vi "host - network - RT (separate).vi"() -> ()   [LabVIEW 2011]
uses:
  Output - Cluster b2g2.ctl
  Input - Cluster b2g2.ctl
panel:
  in  "Pfad":path=path "C:/National Instruments/Logs"
  out "FS-2 [l]":sgl format="%#.2g"
  out "FS-1 [l]":sgl format="%#.2g"
  out "pH-Wert":cluster{"pHS-1":dbl}(graph)
  out "pHS-1":dbl
  in  "Interval [s]":u32=1 min=1 step=1
  in  "Interval [ms]":u32=10 min=10 step=1
  in  "Output - Cluster":T1 {"TS-5 [°C]" format="%#.2g"; "pHS-1 [pH]" format="%.2g"; "TS-4 [°C]" format="%#.2g"; "FS-2 [l]" format="%.2g"; "FS-1 [l]" format="%.2g"; "DS-1 [bar]" format="%#.2g"; "DFS-1 [l/min]" format="%#.2g"; "FS-3 [l]" format="%.2g"; "DFS-1 [dl]" format="%.0g"}
  in  "Host Log":bool
  in  "P-5":bool
  in  "P-5 Drehzahl [%]":u8
  out "T-2 Min!":bool
  out "T-2 Max!":bool
  out "T-1 Min!":bool
  out "T-1 Max!":bool
  in  "Zulauf Füllstandsüberwachung":bool
  in  "MR Füllstandsüberwachung":bool
  out "Heizung":bool
  in  "Temp Soll [°C]":sgl min=0 max=100 step=0.1 format="%.1g"
  in  "Hysterese [°C]":sgl=0.1 min=0.1 max=10 step=0.1 format="%.1g"
  out "Temperaturregelung":cluster{"Temp Soll":sgl, "TS-4":dbl, i32}(graph)
  in  "Temperaturregelung":bool
  out "Temp Ist [°C]":sgl format="%.2g"
  in  "HS-1":bool
  out "Fütterung":bool
  out "Rezikulation":bool
  in  "Zulauf":bool
  out "Dosierung Fertig":bool
  out "Bereits dosiert":sgl
  out "MIN!":bool
  out "MAX!":bool
  out "Pumpendrehzahl":u8
  in  "Dosiermenge [l]":sgl format="%.1g"
  out "Volumen [l]":sgl format="%.1f"
  out "Durchfluss [l/min]":sgl format="%.2f"
  in  "Dosiergeschwindigkeit [l/min]":sgl format="%.1g"
  out "Dosierung":T2(graph)
  in  "Dosierung":bool
  out "Überdruckregelung":cluster{"Druck Soll":sgl, "DS-1":dbl, dbl}(graph)
  in  "Druck Soll [bar]":sgl min=0 max=10 step=0.1 format="%.1g"
  in  "D":sgl
  in  "I":sgl
  in  "P":sgl
  in  "Füllstand Soll [l]":sgl min=0 max=5 step=0.1 format="%.1g"
  in  "D":sgl
  in  "I":sgl
  in  "P":sgl
  in  "Überdruckregelung":bool
  out "Füllstandsregelung":cluster{"Füllstand Soll":sgl, "FS-3":dbl, dbl}(graph)
  in  "Füllstandsregulierung":bool
  in  "P-4":bool
  in  "P-4 Drehzahl  [%]":u8
  in  "Target Log":bool
  in  "V-15  [%]":u8 max=100 step=1
  in  "Input - Cluster":T3 {"Dosiergeschw. [l/min]" format="%.2g"; "Füllstand  P" max=100 step=1 format="%#_3g"; "P-4 Drehzahl [%]" max=100 step=1 format="%#_3g"}
  in  "V-13 [%]":u8 caption="V-13" max=100 step=1
  out "Füllstand Ist":sgl format="%#.2g"
  out "Druck Ist":sgl format="%#.2g"
  in  "stop":bool
  # "Dosierung"
  # "Handsteuerungen"
  # "Max: 4l\nMin: 1l"
  # "T-1"
  # "T-2"
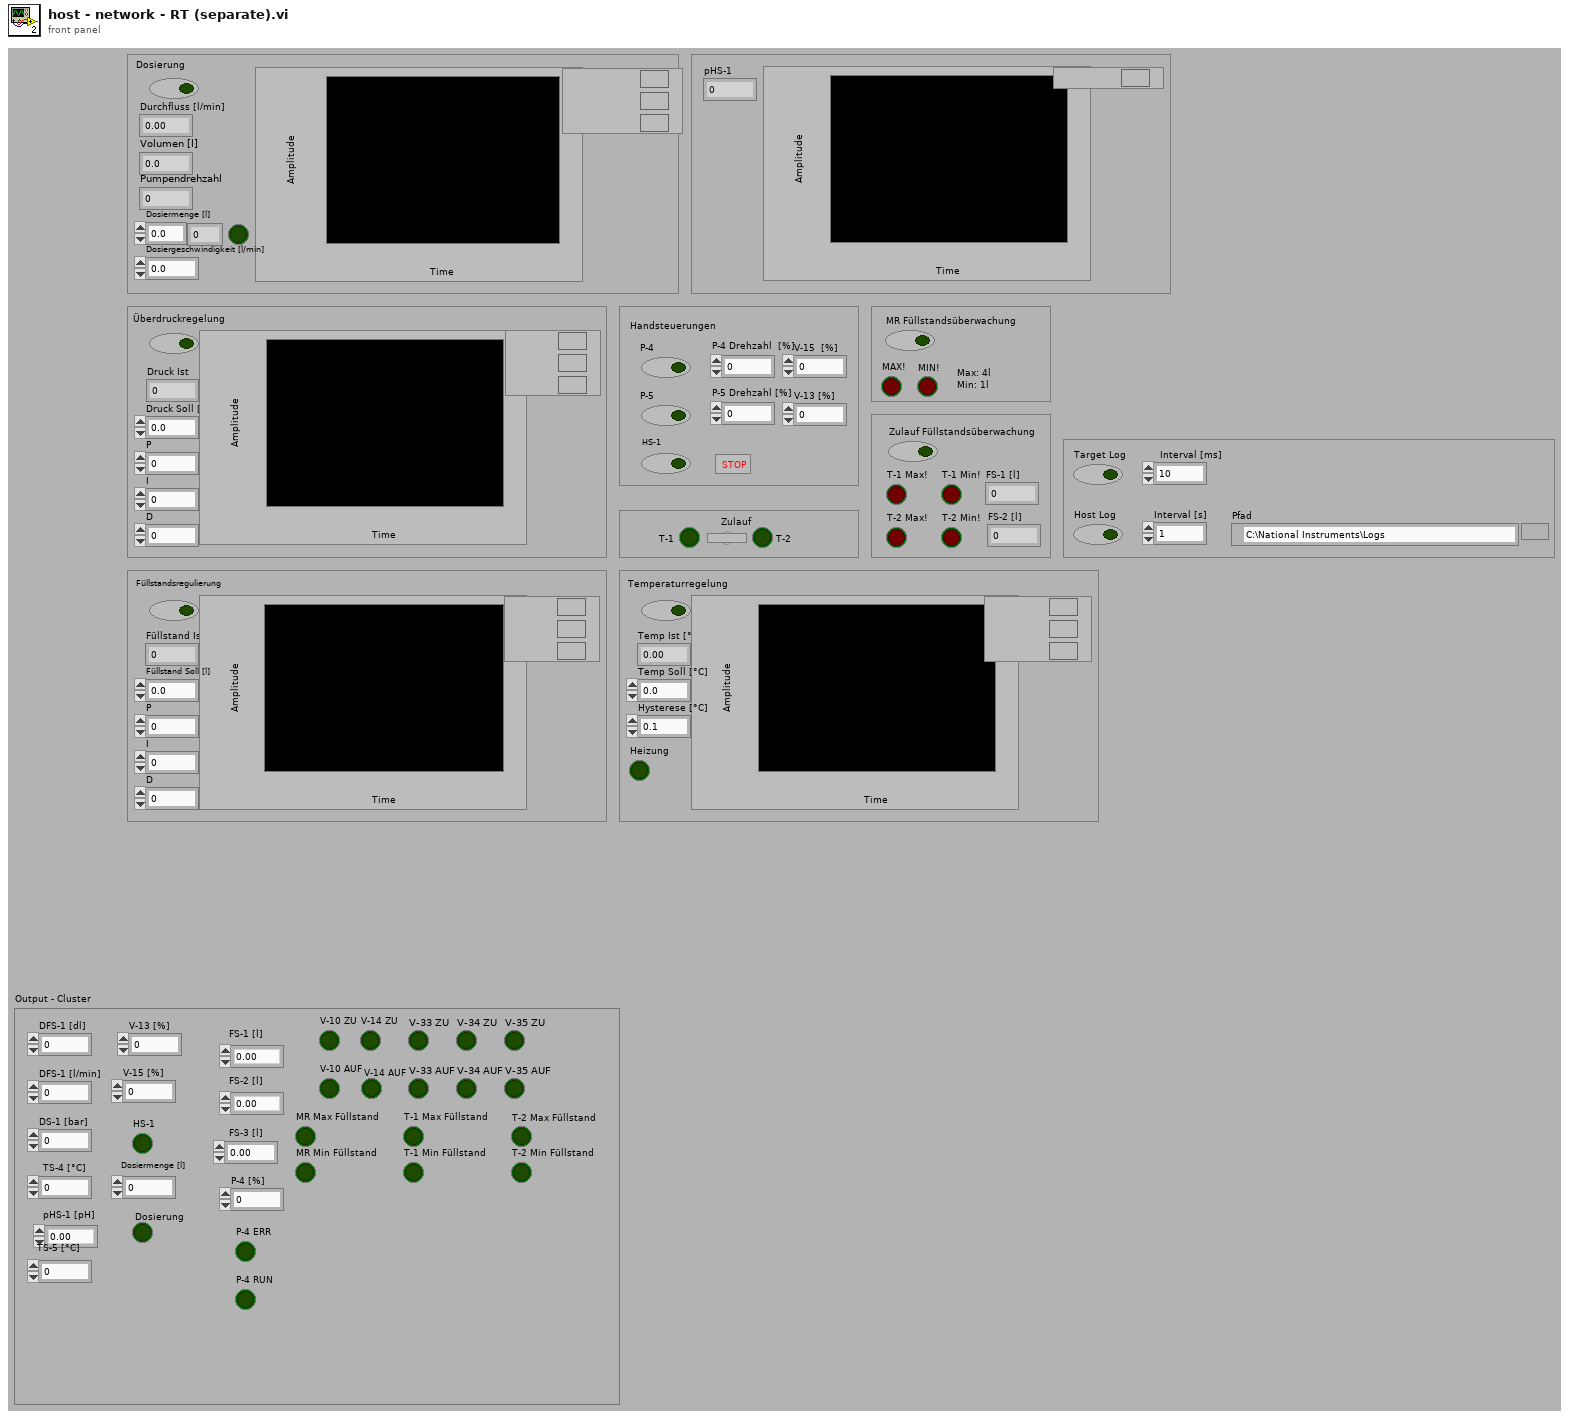
[diagram p1: front panel]
types:
  T1 = typedef "Output - Cluster b2g2.ctl" = cluster{"DFS-1 [dl]":u64, "FS-3 [l]":dbl, "DFS-1 [l/min]":dbl, "DS-1 [bar]":dbl, "V-10 ZU":bool, "V-14 ZU":bool, "FS-1 [l]":dbl, "FS-2 [l]":dbl, "TS-4 [°C]":dbl, "HS-1":bool, "V-13 [%]":u8, "V-15 [%]":u8, "P-4 [%]":u8, "Dosierung":bool, "MR Max Füllstand":bool, "MR Min Füllstand":bool, "Dosiermenge [l]":sgl, "V-14 AUF":bool, "V-10 AUF":bool, "T-1 Max Füllstand":bool, "T-1 Min Füllstand":bool, "T-2 Max Füllstand":bool, "T-2 Min Füllstand":bool, "pHS-1 [pH]":dbl, "P-4 RUN":bool, "V-33 AUF":bool, "V-33 ZU":bool, "V-34 AUF":bool, "V-34 ZU":bool, "P-4 ERR":bool, "TS-5 [°C]":dbl, "V-35 AUF":bool, "V-35 ZU":bool}
  T2 = cluster{"Dosiergeschwindigkeit [l/min]":sgl, "DFS-1 Durchfluss":dbl, dbl}
  T3 = typedef "Input - Cluster b2g2.ctl" = cluster{"V-13 [%]":u8, "V-15 [%]":u8, "Log-Target":bool, "P-4":bool, "P-4 Drehzahl [%]":u8, "Temperaturregelung":bool, "Überdruckregelung":bool, "Füllstandsregulierung":bool, "V-10":bool, "Log-Host":bool, "V-14":bool, "HS-1":bool, "Füllstand  P":sgl, "Füllstand I":sgl, "Füllstand D":sgl, "Füllstand Soll [l]":sgl, "Druck  P":sgl, "Druck I":sgl, "Druck D":sgl, "Druck Soll [bar]":sgl, "Temp Soll [°C]":sgl, "Dosierung":bool, "Dosiermenge [l]":sgl, "Dosiergeschw. [l/min]":sgl, "Tank":bool, "Hysterese [°C]":sgl, "MR Füllstandsüberwachung":bool, "Tank Füllstandsüberwachung":bool, "Log Target [ms]":u32, "Log Host [s]":u32, "Zirkulation EIN [min]":u8, "Zirkulation AUS [min]":u8, "Zirkulation":bool, "V-33":bool, "V-34":bool, "V-35":bool}
  T4 = enum8{"Enabled", "Disabled", "Disabled and Grayed Out"}
  T5 = enum16{"open", "replace", "create", "open or create", "replace or create", "replace or create with confirmation"}
  T6 = cluster{"Temp Soll [°C]":sgl, "TS-4 [°C]":dbl, i32}
  T7 = cluster{"Druck Soll [bar]":sgl, "DS-1 [bar]":dbl, dbl}
  T8 = cluster{"Füllstand Soll [l]":sgl, "FS-3 [l]":dbl, dbl}
  T9 = cluster{"Dosiergeschwindigkeit [l/min]":sgl, "DFS-1 [l/min]":dbl, dbl}
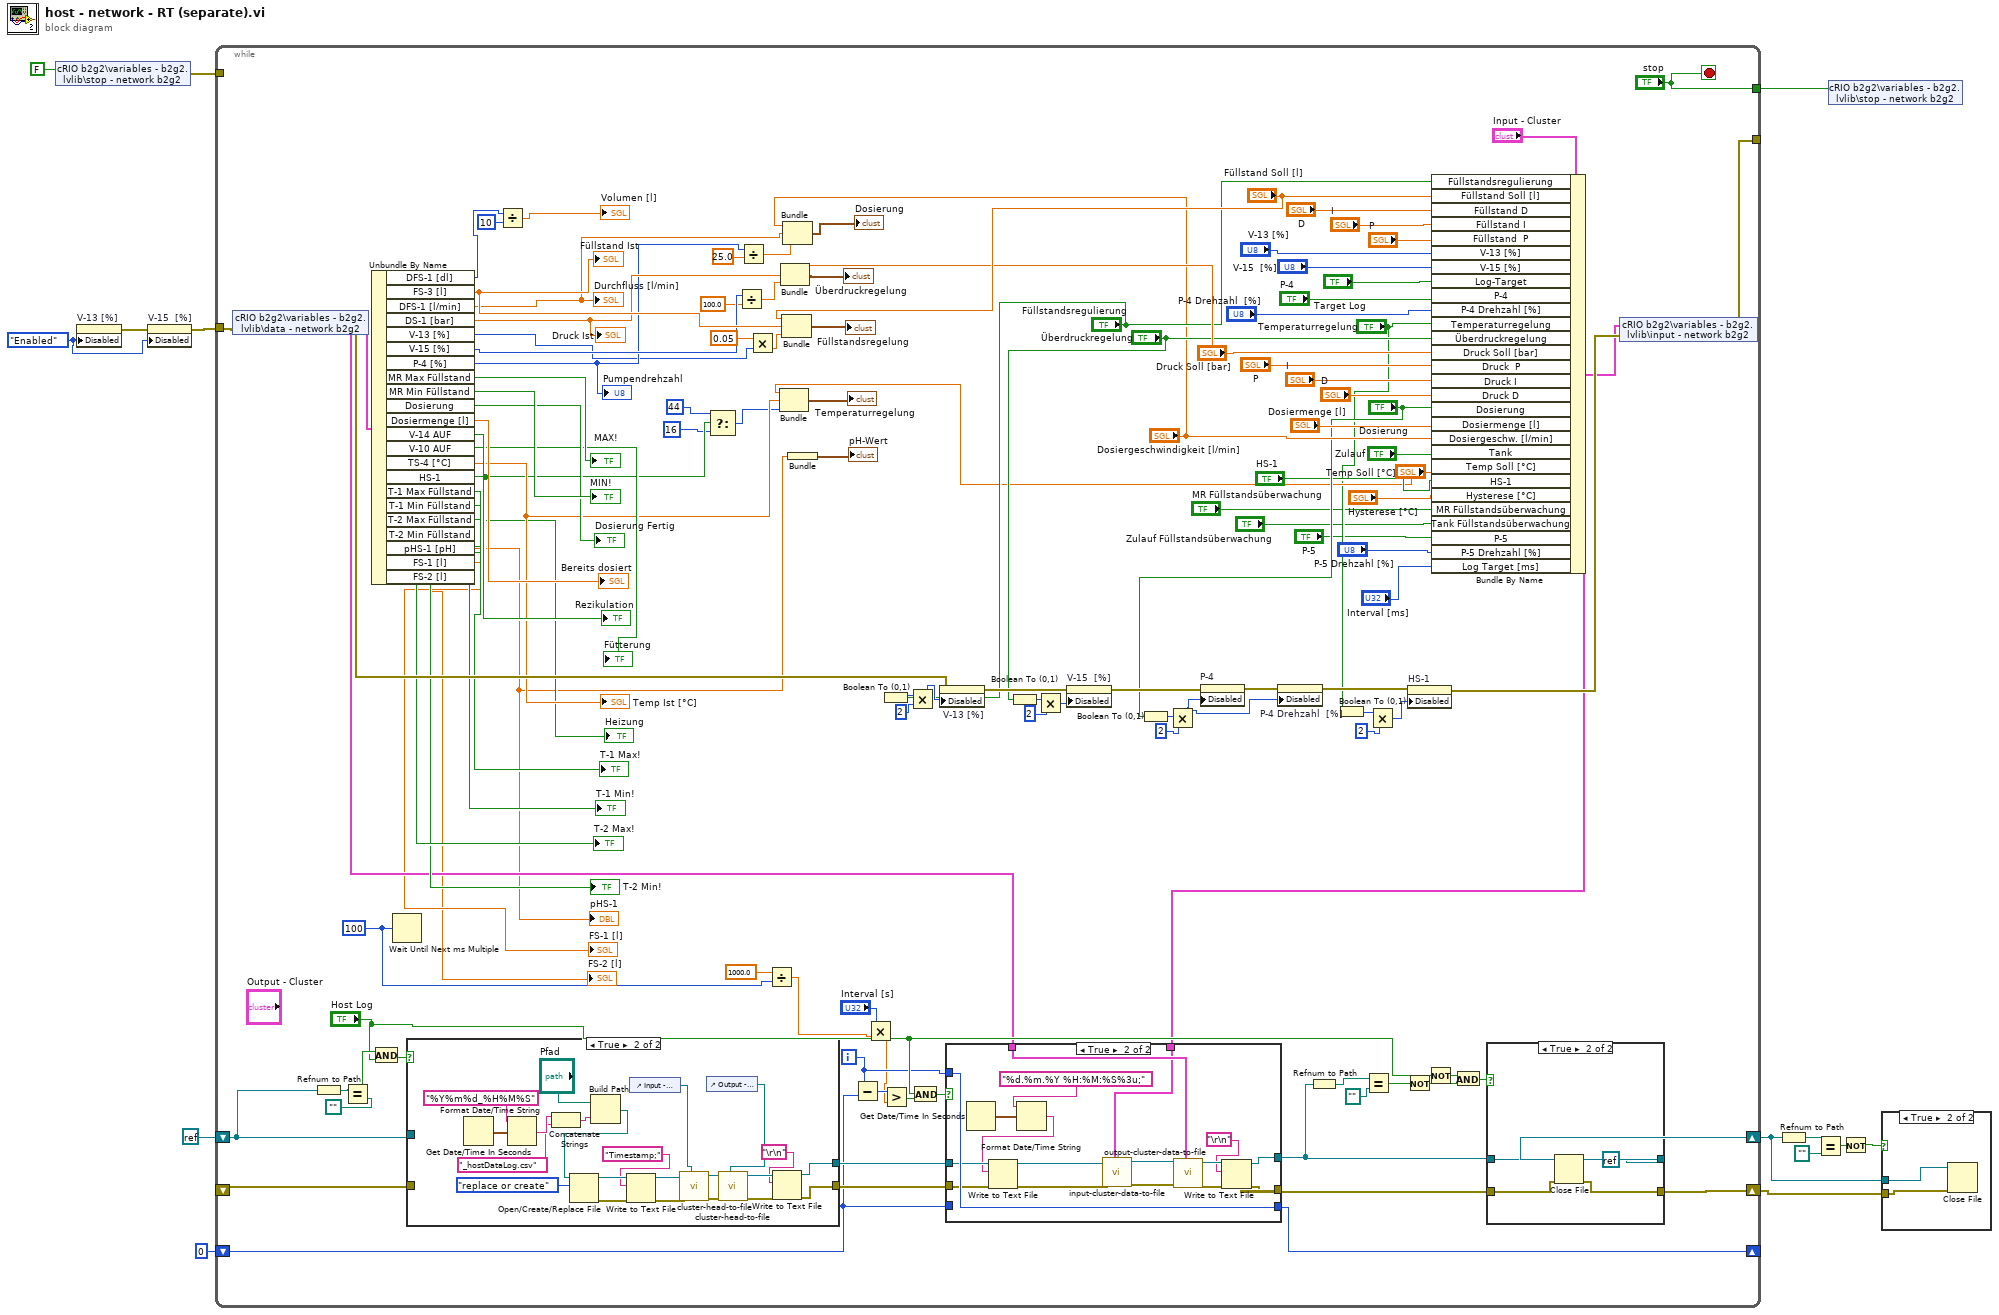
[diagram p0: block diagram]
diagram:
  w10 = T4."Enabled" ("Disabled")
  n1 = shared-variable "cRIO b2g2\\variables - b2g2.lvlib\\stop - network b2g2"(FALSE) -> (error out=w13:errorcluster)  [unwired: 1 in]
  n2 = property on="V-13 [%]" class="DigNum (strict)"("Disabled"=w10) -> (error out=w11:errorcluster)  [unwired: 2 in, 1 out]
  n3 = property on="V-15  [%]" class="DigNum (strict)"(error in=w11, "Disabled"=w10) -> (error out=w9:errorcluster)  [unwired: 1 in, 1 out]
  n4 = while {
    tunnel: ["stop"] -> w14
    tunnel: w13 -> [_]
    tunnel: [w93] -> _
    tunnel: w9 -> [w59]
    shift-right: [w41] -> w4
    shift-left: refnum<k0> refnum -> [w38]
    shift-right: [w40] -> w3
    shift-left: _ -> [w39]
    shift-right: [w34] -> _
    shift-left: 0 -> [w35]
    i -> [w36]
    stop <- "stop" stop-if-true
    w28 = u32 100 ("millisecond multiple")
    n5 = shared-variable "cRIO b2g2\\variables - b2g2.lvlib\\data - network b2g2"(error in=w59) -> (w33:T1, error out=w94:errorcluster)
    n6 = Refnum to Path(1:w38) -> (0:w45:path)
    n7 = Equal?(x=w45, y=path "") -> (x = y?=w42:bool)
    n8 = Unbundle By Name(w33) -> ("DFS-1 [dl]"=w100:u64, "FS-3 [l]"=w128:dbl, "DFS-1 [l/min]"=w103:dbl, "DS-1 [bar]"=w119:dbl, "V-13 [%]"=w15:u8, "V-15 [%]"=w116:u8, "P-4 [%]"=w96:u8, "MR Max Füllstand"=→"MAX!":bool, "MR Min Füllstand"=→"MIN!":bool, "Dosierung"=→"Dosierung Fertig":bool, "Dosiermenge [l]"=→"Bereits dosiert":sgl, "V-14 AUF"=→"Rezikulation":bool, "V-10 AUF"=→"Fütterung":bool, "TS-4 [°C]"=w78:dbl, "HS-1"=w75:bool, "T-1 Max Füllstand"=→"T-1 Max!":bool, "T-1 Min Füllstand"=→"T-1 Min!":bool, "T-2 Max Füllstand"=→"T-2 Max!":bool, "T-2 Min Füllstand"=→"T-2 Min!":bool, "pHS-1 [pH]"=w21:dbl, "FS-1 [l]"=→"FS-1 [l]":dbl, "FS-2 [l]"=→"FS-2 [l]":dbl)
    "Füllstand Ist" <- w128
    "Durchfluss [l/min]" <- w103
    "Druck Ist" <- w119
    "Pumpendrehzahl" <- w96
    "Temp Ist [°C]" <- w78
    "Heizung" <- w75
    "pHS-1" <- w21
    n9 = And(x=w42, y="Host Log") -> (x .and. y?=w43:bool)
    n10 = Wait Until Next ms Multiple(millisecond multiple=w28) -> ()  [unwired: 1 out]
    n11 = case shown="True" w43 {
      tunnel: [w135 w144] -> w47
      tunnel: [w136 w143] -> w46
      tunnel: w39 -> [w136 _]
      tunnel: w38 -> [w135 _]
      frame False {
      }
      frame True {
        n12 = Get Date/Time In Seconds() -> (seconds since 1Jan1904=w156:timestamp)
        n13 = Format Date/Time String(time format string (%c)="%Y%m%d_%H%M%S", seconds (now)=w156) -> (date/time string=w155:string)  [unwired: 1 in]
        n14 = Concatenate Strings(w155, "_hostDataLog.csv" ("name or relative path")) -> (w152:string)
        n15 = Build Path(base path="Pfad", name or relative path=w152) -> (appended path=w151:path)
        n16 = Open/Create/Replace File(file path (use dialog)=w151, operation (0:open)=T5."replace or create") -> (refnum out=w141:refnum<file>, error out=w140:errorcluster)  [unwired: 4 in, 1 out]
        n17 = Write to Text File(file (use dialog)=w141, text="Timestamp;", error in=w140) -> (refnum out=w138:refnum<file>, error out=w139:errorcluster)  [unwired: 1 in, 1 out]
        n18 = control-ref of="Input - Cluster"() -> (w147:refnum<vi>)
        n19 = call "cluster-head-to-file.vi"("refnum in"=w138, "error in"=w139, "cluster ref"=w147) -> ("refnum out"=w149:refnum<file>, "error out"=w148:errorcluster)  [unwired: 6 in]
        n20 = control-ref of="Output - Cluster"() -> (w150:refnum<vi>)
        n21 = call "cluster-head-to-file.vi"("refnum in"=w149, "error in"=w148, "cluster ref"=w150) -> ("refnum out"=w146:refnum<file>, "error out"=w145:errorcluster)  [unwired: 6 in]
        n22 = Write to Text File(file (use dialog)=w146, text="\r\n", error in=w145) -> (refnum out=w144:refnum<file>, error out=w143:errorcluster)  [unwired: 1 in, 1 out]
      }
    }
    n23 = Divide(x=w100, y=u64 10) -> (x/y=→"Volumen [l]":dbl)
    n24 = Select(t=44, s=w75, f=16) -> (s? t:f=w25:i32)
    n25 = Divide(x=w116, y=100.0) -> (x/y=w117:dbl)
    n26 = Divide(x=w96, y=25.0) -> (x/y=w97:dbl)
    n27 = Multiply(x=0.05, y=w15) -> (x*y=w17:dbl)
    n28 = Divide(x=1000.0, y=w28) -> (x/y=w27:dbl)
    n29 = Bundle("Temp Soll [°C]"="Temp Soll [°C]", "TS-4 [°C]"=w78, w25) -> (→"Temperaturregelung":T6)  [unwired: 1 in]
    n30 = Bundle("Druck Soll [bar]"="Druck Soll [bar]", "DS-1 [bar]"=w119, w117) -> (→"Überdruckregelung":T7)  [unwired: 1 in]
    n31 = Bundle("Füllstand Soll [l]"="Füllstand Soll [l]", "FS-3 [l]"=w128, w17) -> (→"Füllstandsregelung":T8)  [unwired: 1 in]
    n32 = Bundle("Dosiergeschwindigkeit [l/min]"="Dosiergeschwindigkeit [l/min]", "DFS-1 [l/min]"=w103, w97) -> (→"Dosierung":T9)  [unwired: 1 in]
    n33 = Bundle("pHS-1 [pH]"=w21) -> (→"pH-Wert":cluster{"pHS-1 [pH]":dbl})  [unwired: 1 in]
    n34 = Subtract(x=w36, y=w35) -> (x-y=w58:i32)
    n35 = Multiply(x="Interval [s]", y=w27) -> (x*y=w31:dbl)
    n36 = Boolean To (0,1)(Boolean="Füllstandsregulierung") -> (0, 1=w110:i16)
    n37 = Greater?(x=w58, y=w31) -> (0:w57:bool)
    n38 = Multiply(x=w110, y=i16 2) -> (x*y=w108:i16)
    n39 = And(x="Host Log", y=w57) -> (x .and. y?=w56:bool)
    n40 = property on="V-13 [%]" class="DigNum (strict)"(error in=w94, "Disabled"=w108) -> (error out=w112:errorcluster)  [unwired: 1 in, 1 out]
    n41 = Boolean To (0,1)(Boolean="Überdruckregelung") -> (0, 1=w106:i16)
    n42 = Multiply(x=w106, y=i16 2) -> (x*y=w107:i16)
    n43 = property on="V-15  [%]" class="DigNum (strict)"(error in=w112, "Disabled"=w107) -> (error out=w92:errorcluster)  [unwired: 1 in, 1 out]
    n44 = Boolean To (0,1)(Boolean="Dosierung") -> (0, 1=w89:i16)
    n45 = Multiply(x=w89, y=i16 2) -> (x*y=w87:i16)
    n46 = property on="P-4" class="Bool (strict)"(error in=w92, "Disabled"=w87) -> (error out=w91:errorcluster)  [unwired: 1 in, 1 out]
    n47 = property on="P-4 Drehzahl  [%]" class="DigNum (strict)"(error in=w91, "Disabled"=w87) -> (error out=w74:errorcluster)  [unwired: 1 in, 1 out]
    n48 = Boolean To (0,1)(Boolean="Temperaturregelung") -> (0, 1=w70:i16)
    n49 = Multiply(x=w70, y=i16 2) -> (x*y=w69:i16)
    n50 = property on="HS-1" class="Bool (strict)"(error in=w74, "Disabled"=w69) -> (error out=w73:errorcluster)  [unwired: 1 in, 1 out]
    n51 = Not(x="Host Log") -> (.not. x?=w49:bool)
    n52 = Bundle By Name(cluster="Input - Cluster", "Füllstandsregulierung"="Füllstandsregulierung", "Füllstand Soll [l]"="Füllstand Soll [l]", "Füllstand D"="D", "Füllstand I"="I", "Füllstand  P"="P", "V-13 [%]"="V-13 [%]", "V-15 [%]"="V-15  [%]", "Log-Target"="Target Log", "P-4"="P-4", "P-4 Drehzahl [%]"="P-4 Drehzahl  [%]", "Temperaturregelung"="Temperaturregelung", "Überdruckregelung"="Überdruckregelung", "Druck Soll [bar]"="Druck Soll [bar]", "Druck  P"="P", "Druck I"="I", "Druck D"="D", "Dosierung"="Dosierung", "Dosiermenge [l]"="Dosiermenge [l]", "Dosiergeschw. [l/min]"="Dosiergeschwindigkeit [l/min]", "Tank"="Zulauf", "Temp Soll [°C]"="Temp Soll [°C]", "HS-1"="HS-1", "Hysterese [°C]"="Hysterese [°C]", "MR Füllstandsüberwachung"="MR Füllstandsüberwachung", "Tank Füllstandsüberwachung"="Zulauf Füllstandsüberwachung", "P-5"="P-5", "P-5 Drehzahl [%]"="P-5 Drehzahl [%]", "Log Target [ms]"="Interval [ms]") -> (w32:T3)
    n53 = case shown="True" w56 {
      tunnel: [w166 w181] -> w53
      tunnel: [w167 w179] -> w55
      tunnel: w47 -> [w166 w177]
      tunnel: w46 -> [w167 w176]
      tunnel: w36 -> [_ w184]
      tunnel: w35 -> [w165 _]
      tunnel: [w165 w184] -> w34
      tunnel: w33 -> [_ w183]
      tunnel: w32 -> [_ w168]
      frame False {
      }
      frame True {
        n54 = Get Date/Time In Seconds() -> (seconds since 1Jan1904=w175:timestamp)
        n55 = Format Date/Time String(time format string (%c)="%d.%m.%Y %H:%M:%S%3u;", seconds (now)=w175) -> (date/time string=w173:string)  [unwired: 1 in]
        n56 = Write to Text File(file (use dialog)=w177, text=w173, error in=w176) -> (refnum out=w170:refnum<file>, error out=w169:errorcluster)  [unwired: 1 in, 1 out]
        n57 = call "input-cluster-data-to-file.vi"("refnum in"=w170, "error in"=w169, "Input - Cluster"=w168) -> ("refnum out"=w172:refnum<file>, "error out"=w171:errorcluster)  [unwired: 6 in]
        n58 = call "output-cluster-data-to-file.vi"("refnum in"=w172, "error in"=w171, "Output - Cluster"=w183) -> ("refnum out"=w182:refnum<file>, "error out"=w180:errorcluster)  [unwired: 6 in]
        n59 = Write to Text File(file (use dialog)=w182, text="\r\n", error in=w180) -> (refnum out=w181:refnum<file>, error out=w179:errorcluster)  [unwired: 1 in, 1 out]
      }
    }
    n60 = Refnum to Path(1:w53) -> (0:w52:path)
    n61 = Equal?(x=w52, y=path "") -> (x = y?=w50:bool)
    n62 = Not(x=w50) -> (.not. x?=w48:bool)
    n63 = And(x=w49, y=w48) -> (x .and. y?=w54:bool)
    n64 = case shown="True" w54 {
      tunnel: [w160 refnum<k0> refnum] -> w41
      tunnel: w53 -> [w160 w164]
      tunnel: [w159 w162] -> w40
      tunnel: w55 -> [w159 w163]
      frame False {
      }
      frame True {
        n65 = Close File(refnum=w164, error in=w163) -> (error out=w162:errorcluster)  [unwired: 1 out]
      }
    }
    n66 = shared-variable "cRIO b2g2\\variables - b2g2.lvlib\\input - network b2g2"(w32, error in=w73) -> (error out=w93:errorcluster)
  }
  n67 = Refnum to Path(1:w4) -> (0:w6:path)
  n68 = Equal?(x=w6, y=path "") -> (x = y?=w8:bool)
  n69 = shared-variable "cRIO b2g2\\variables - b2g2.lvlib\\stop - network b2g2"(w14) -> ()  [unwired: 1 in, 1 out]
  n70 = Not(x=w8) -> (.not. x?=w7:bool)
  n71 = case shown="True" w7 {
    tunnel: w4 -> [_ w186]
    tunnel: w3 -> [_ w185]
    frame False {
    }
    frame True {
      n72 = Close File(refnum=w186, error in=w185) -> ()  [unwired: 2 out]
    }
  }
